vi "Set Settings Visibility.vi"(8 "error in (no error)":errorcluster, 10 "Visible":bool, 11 "UI Controller in":refnum<class "UI Controller.lvclass">) -> (0 "error out":errorcluster, 3 "UI Controller out":refnum<class "UI Controller.lvclass">)   [LabVIEW 2020, in "UI Controller.lvlib" / "UI Controller.lvclass"]
uses:
  UI Controller.lvclass
  C:/Program Files/National Instruments/LabVIEW 2020/vi.lib/ActorFrameworkMVC/View Controller/View Controller/View Controller.lvclass
  <vilib>/Utility/miscctls.llb/LVPositionTypeDef.ctl
  <vilib>/ActorFrameworkMVC/View Controller/View Controller/View Controller.lvclass
panel:
  # "NOTICE -- YOU MUST LEAVE THIS NOTICE IN PLACE.\n\nCopyright (c) 2017, LIANG LIU Shawn.Liu.cn@gmail.com\nAll rights reserved.\n\nRedistribution and use in source and binary forms, with or without modification, are permitted provided that the following conditions are met:\n-Redistributions of source code must retain the above copyright notice, this list of conditions and the following disclaimer.\n-Redistributions in binary form must reproduce the above copyright notice, this list of conditions and the following disclaimer in the documentation and/or other materials provided with the distribution.\n-Neither the name of the eLp nor the names of its contributors may be used to endorse or promote products derived from this software without specific prior written permission.\n\nTHIS SOFTWARE IS PROVIDED BY THE COPYRIGHT HOLDERS AND CONTRIBUTORS \"AS IS\" AND ANY EXPRESS OR IMPLIED WARRANTIES, INCLUDING, BUT NOT LIMITED TO, THE IMPLIED WARRANTIES OF MERCHANTABILITY AND FITNESS FOR A PARTICULAR PURPOSE ARE DISCLAIMED. IN NO EVENT SHALL THE COPYRIGHT HOLDER OR CONTRIBUTORS BE LIABLE FOR ANY DIRECT, INDIRECT, INCIDENTAL, SPECIAL, EXEMPLARY, OR CONSEQUENTIAL DAMAGES (INCLUDING, BUT NOT LIMITED TO, PROCUREMENT OF SUBSTITUTE GOODS OR SERVICES; LOSS OF USE, DATA, OR PROFITS; OR BUSINESS INTERRUPTION) HOWEVER CAUSED AND ON ANY THEORY OF LIABILITY, WHETHER IN CONTRACT, STRICT LIABILITY, OR TORT (INCLUDING NEGLIGENCE OR OTHERWISE) ARISING IN ANY WAY OUT OF THE USE OF THIS SOFTWARE, EVEN IF ADVISED OF THE POSSIBILITY OF SUCH DAMAGE."
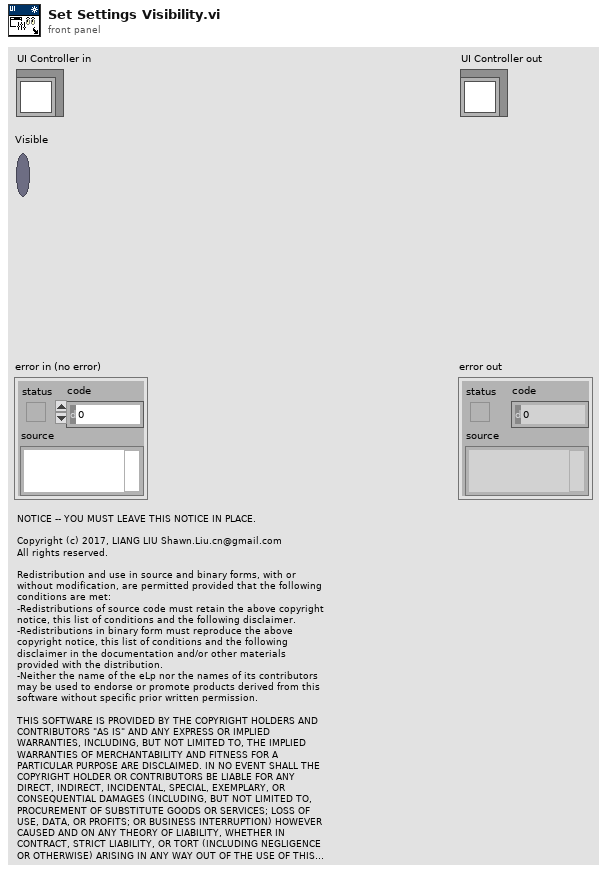
[diagram p1: front panel]
types:
  T1 = typedef "LVPositionTypeDef.ctl" = cluster{"Left":i32, "Top":i32}
  T2 = typedef "LVBoundsTypeDef.ctl" = cluster{"Width":u32, "Height":u32}
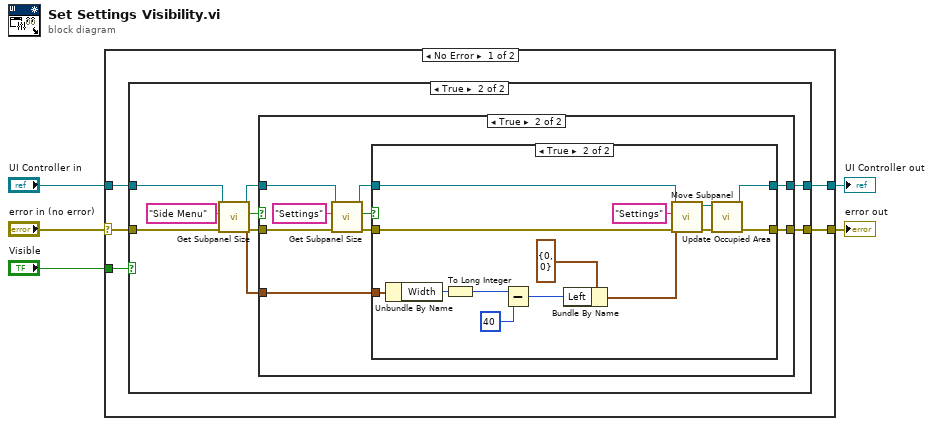
[diagram p0: block diagram]
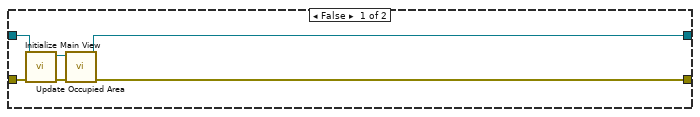
[diagram p2: hidden frame]
diagram:
  n1 = case shown="No Error" "error in (no error)" {
    selector: "error in (no error)" -> [w6 w54]
    tunnel: [w10 w54] -> w5
    tunnel: [w9 w53] -> w4
    tunnel: "UI Controller in" -> [w8 w53]
    tunnel: "Visible" -> [w7 _]
    frame No Error {
      n2 = case shown="True" w7 {
        tunnel: [w13 w25] -> w10
        tunnel: [w11 w24] -> w9
        tunnel: w8 -> [w14 w23]
        tunnel: w6 -> [w16 w17]
        frame False {
          n3 = call "Initialize Main View.vi"("error in (no error)"=w16, "UI Controller in"=w14) -> ("error out"=w15:errorcluster, "UI Controller out"=w12:refnum<class "UI Controller.lvclass">)  [unwired: 8 in]
          n4 = call "Update Occupied Area.vi"("error in (no error)"=w15, "UI Controller in"=w12) -> ("error out"=w13:errorcluster, "UI Controller out"=w11:refnum<class "UI Controller.lvclass">)  [unwired: 8 in]
        }
        frame True {
          n5 = call <vilib>:"Get Subpanel Size.vi"("error in (no error)"=w17, "Subpanel Name"="Side Menu", "View Controller in"=w23) -> ("error out"=w22:errorcluster, "Subpanel Size"=w18:T2, "Found?"=w20:bool, "View Controller out"=w19:refnum<class "UI Controller.lvclass">)  [unwired: 5 in]
          n6 = case shown="True" w20 {
            tunnel: [w27 w29] -> w25
            tunnel: [w26 w30] -> w24
            tunnel: w22 -> [w27 w36]
            tunnel: w19 -> [w26 w35]
            tunnel: w18 -> [_ w28]
            frame False {
            }
            frame True {
              n7 = call <vilib>:"Get Subpanel Size.vi"("error in (no error)"=w36, "Subpanel Name"="Settings", "View Controller in"=w35) -> ("error out"=w33:errorcluster, "Found?"=w31:bool, "View Controller out"=w32:refnum<class "UI Controller.lvclass">)  [unwired: 5 in, 1 out]
              n8 = case shown="True" w31 {
                tunnel: [w38 w48] -> w29
                tunnel: [w37 w46] -> w30
                tunnel: w33 -> [w38 w50]
                tunnel: w32 -> [w37 w49]
                tunnel: w28 -> [_ w44]
                frame False {
                }
                frame True {
                  n9 = Unbundle By Name(w44) -> ("Width"=w45:u32)
                  n10 = To Long Integer(number=w45) -> (32bit integer=w41:i32)
                  n11 = Subtract(x=w41, y=40) -> (x-y=w42:i32)
                  n12 = Bundle By Name(cluster=T1 {"Left"=0, "Top"=0} ("Position"), "Left"=w42) -> (w39:T1)
                  n13 = call-dynamic "Move Subpanel.vi"("error in (no error)"=w50, "Position"=w39, "Subpanel Name"="Settings", "View Controller in"=w49) -> ("error out"=w51:errorcluster, "View Controller out"=w47:refnum<class "UI Controller.lvclass">)  [unwired: 6 in]
                  n14 = call "Update Occupied Area.vi"("error in (no error)"=w51, "UI Controller in"=w47) -> ("error out"=w48:errorcluster, "UI Controller out"=w46:refnum<class "UI Controller.lvclass">)  [unwired: 8 in]
                }
              }
            }
          }
        }
      }
    }
    frame Error {
    }
  }
  "error out" <- w5
  "UI Controller out" <- w4
